vi "ma_SML ND Zoom FFT (real input).vi"(4 "error in (no error)":errorcluster, 5 "zoom FFT settings":T1={"zoom settings"={"center frequency"=-inf, "zoom"=1, "trim"=1.0}, "FFT settings"={"window"=1, "FFT size"=-1}} {"FFT settings"."window" items=["Rectangle"=0, "Hanning"=1, "Hamming"=2, "Blackman-Harris"=3, "Exact Blackman"=4, "Blackman"=5, "Flat Top"=6, "4 Term B-Harris "=7, "7 Term B-Harris"=8, "Low Sidelobe"=9, "Blackman Nuttall"=11, "Triangle"=30, "Bartlett-Hanning"=31, "Bohman"=32, "Parzen"=33, "Welch"=34, "Kaiser"=60, "Dolph-Chebyshev"=61, "Gaussian"=62]; "zoom settings"."trim" min=1.0 format="%.2f"; "zoom settings"."center frequency" format="%.2f"; "zoom settings"."zoom" min=1}, 6 "fs":dbl=1024.0 format="%.2f", 7 "x":dbl[](array[numeric]) format="%.2f") -> (0 "error out":errorcluster, 2 "spectral info":T2 {"window" items=["Rectangle"=0, "Hanning"=1, "Hamming"=2, "Blackman-Harris"=3, "Exact Blackman"=4, "Blackman"=5, "Flat Top"=6, "4 Term B-Harris "=7, "7 Term B-Harris"=8, "Low Sidelobe"=9, "Blackman Nuttall"=11, "Triangle"=30, "Bartlett-Hanning"=31, "Bohman"=32, "Parzen"=33, "Welch"=34, "Kaiser"=60, "Dolph-Chebyshev"=61, "Gaussian"=62]}, 3 "FFT spectrum[Vrms]":T3={"f0"=0.0, "df"=1.0, "spectrum"=[]} {"spectrum" format="%.2f"; "df" format="%.2f"; "f0" format="%.2f"})   [LabVIEW 2020, in "NI_MAPro.lvlib"]
uses:
  NI_MAPro.lvlib
  ma_sml_Spectrum Cluster (complex).ctl
  ma_sml_Spectral Info.ctl
  ma_sml_ND Zoom FFT Settings.ctl
  NI_AALPro.lvlib
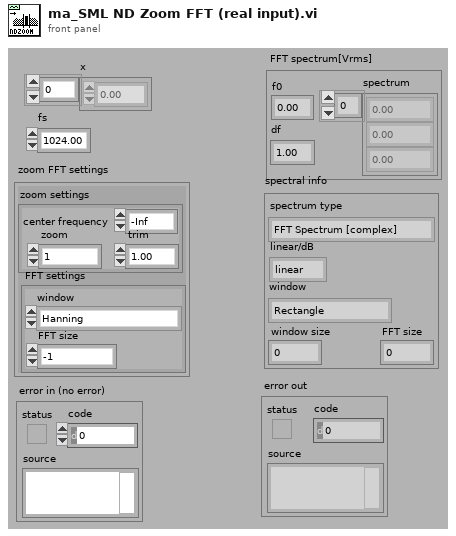
[diagram p1: front panel]
types:
  T1 = typedef "NI_MAPro.lvlib/ma_sml_ND Zoom FFT Settings.ctl" = cluster{"zoom settings":cluster{"center frequency":dbl, "zoom":i32, "trim":dbl}, "FFT settings":cluster{"window":u16, "FFT size":i32}}
  T2 = typedef "NI_MAPro.lvlib/ma_sml_Spectral Info.ctl" = cluster{"spectrum type":enum16{"FFT Spectrum [complex]", "Amplitude [Magnitude]", "Power [Magnitude^2]", "Cross Spectrum [complex]", "Frequency Response [Complex]"}, "linear/dB":enum16{"linear", "dB"}, "window":u16, "window size":i32, "FFT size":i32}
  T3 = typedef "NI_MAPro.lvlib/ma_sml_Spectrum Cluster (complex).ctl" = cluster{"f0":dbl, "df":dbl, "spectrum":cdb[]}
  T4 = cluster{"center frequency":dbl, "zoom":i32, "trim":dbl}
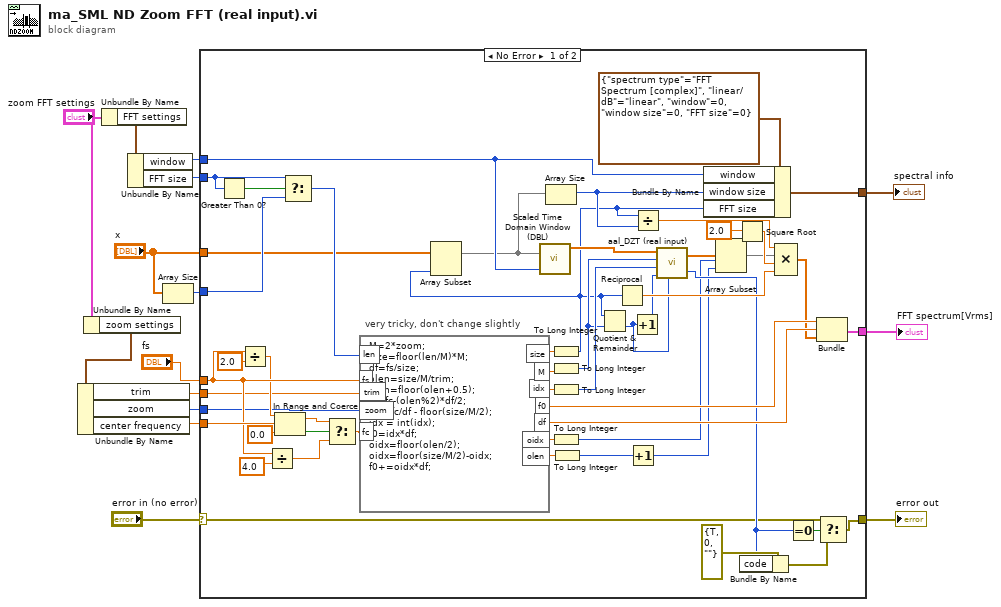
[diagram p0: block diagram]
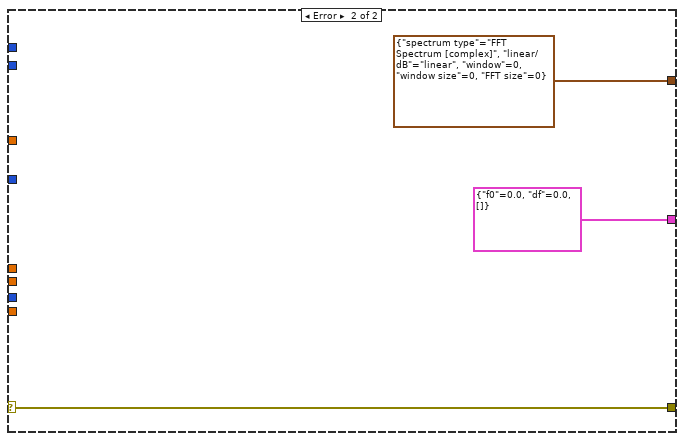
[diagram p2: hidden frame]
diagram:
  n1 = Unbundle By Name("zoom FFT settings") -> ("zoom settings"=w4:T4)
  n2 = Unbundle By Name(w4) -> ("trim"=w1:dbl, "zoom"=w2:i32, "center frequency"=w13:dbl)
  n3 = Unbundle By Name("zoom FFT settings") -> ("FFT settings"=w6:cluster{"window":u16, "FFT size":i32})
  n4 = Unbundle By Name(w6) -> ("window"=w8:u16, "FFT size"=w9:i32)
  n5 = Array Size(array="x") -> (size(s)=w7:i32)
  n6 = case shown="No Error" "error in (no error)" {
    selector: "error in (no error)" -> [w17 w69]
    tunnel: "x" -> [w19 _]
    tunnel: "fs" -> [w35 _]
    tunnel: [w67 cluster{"f0":dbl, "df":dbl, cdb[]} {"f0"=0.0, "df"=0.0, []}] -> w11
    tunnel: [w60 w69] -> w15
    tunnel: w2 -> [w22 _]
    tunnel: w13 -> [w36 _]
    tunnel: [w53 T2 {"spectrum type"=enum."FFT Spectrum [complex]", "linear/dB"=enum."linear", "window"=0, "window size"=0, "FFT size"=0} ("spectral info")] -> w12
    tunnel: w8 -> [w46 _]
    tunnel: w9 -> [w31 _]
    tunnel: w7 -> [w30 _]
    tunnel: w1 -> [w21 _]
    frame No Error {
      # "very tricky, don't change slightly"
      n7 = Greater Than 0?(x=w31) -> (x > 0?=w45:bool)
      n8 = Divide(x=w35, y=2.0) -> (x/y=w33:dbl)
      n9 = Divide(x=w35, y=4.0) -> (x/y=w54:dbl)
      n10 = In Range and Coerce(upper limit=w33, x=w36, lower limit=0.0) -> (coerced(x)=w23:dbl, In Range?=w37:bool)
      n11 = Select(t=w31, s=w45, f=w30) -> (s? t:f=w29:i32)
      n12 = Select(t=w23, s=w37, f=w54) -> (s? t:f=w56:dbl)
      n13 = formula code="M=2*zoom;\nsize=floor(len/M)*M;\ndf=fs/size;\nolen=size/M/trim;\nolen=floor(olen+0.5);\nfc=fc-(olen%2)*df/2;\nidx=fc/df - floor(size/M/2);\nidx = int(idx);\nf0=idx*df;\noidx=floor(olen/2);\noidx=floor(size/M/2)-oidx;\nf0+=oidx*df;"("fs"=w35, "fc"=w56, "zoom"=w22, "len"=w29, "trim"=w21) -> ("f0"=w64:dbl, "df"=w63:dbl, "idx"=w50:dbl, "size"=w49:dbl, "M"=w51:dbl, "oidx"=w42:dbl, "olen"=w41:dbl)
      n14 = To Long Integer(number=w49) -> (32bit integer=w18:i32)
      n15 = Array Subset(array=w19, length=w18) -> (w20:dbl[])  [unwired: 1 in]
      n16 = call "Scaled Time Domain Window (DBL).vi"("window"=w46, "X"=w20) -> ("Windowed X"=w52:dbl[])  [unwired: 7 in, 2 out]
      n17 = Array Size(array=w20) -> (size(s)=w27:i32)
      n18 = To Long Integer(number=w51) -> (32bit integer=w47:i32)
      n19 = To Long Integer(number=w50) -> (32bit integer=w48:i32)
      n20 = To Long Integer(number=w42) -> (32bit integer=w39:i32)
      n21 = To Long Integer(number=w41) -> (32bit integer=w38:i32)
      n22 = Quotient & Remainder(x=w18, y=w47) -> (floor(x/y)=w24:i32)  [unwired: 1 out]
      n23 = Reciprocal(x=w18) -> (1/x=w57:dbl)
      n24 = Increment(x=w38) -> (x+1=w26:i32)
      n25 = Increment(x=w24) -> (x+1=w25:i32)
      n26 = Divide(x=w18, y=w27) -> (x/y=w28:dbl)
      n27 = call "aal_DZT (real input).vi"("x"=w52, "M"=w47, "index"=w48, "out_len"=w25, "fft_len"=w24) -> ("Y"=w43:cdb[], "error"=w40:i32)
      n28 = Bundle By Name(cluster=T2 {"spectrum type"=enum."FFT Spectrum [complex]", "linear/dB"=enum."linear", "window"=0, "window size"=0, "FFT size"=0} ("spectral info"), "window"=w46, "window size"=w27, "FFT size"=w18) -> (w53:T2)
      n29 = Array Subset(array=w43, index=w39, length=w26) -> (w44:cdb[])
      n30 = Square Root(x=2.0) -> (sqrt(x)=w65:dbl)
      n31 = Bundle By Name(cluster=errorcluster {"status"=TRUE, "code"=0, "source"=""} ("error in (no error)"), "code"=w40) -> (w58:errorcluster)
      n32 = Compound Arithmetic op=MULTIPLY(w28, w44, w65, w57) -> (w62:cdb[])
      n33 = Equal To 0?(x=w40) -> (x = 0?=w61:bool)
      n34 = Bundle("f0"=w64, "df"=w63, w62) -> (w67:cluster{"f0":dbl, "df":dbl, cdb[]})  [unwired: 1 out]
      n35 = Select(t=w17, s=w61, f=w58) -> (s? t:f=w60:errorcluster)
    }
    frame Error {
    }
  }
  "FFT spectrum[Vrms]" <- w11
  "error out" <- w15
  "spectral info" <- w12
